vi "Create temperature log file.vi"(4 "path in":path) -> (0 "error out":errorcluster, 1 "refnum out":refnum<file>)   [LabVIEW 2022 SP3]
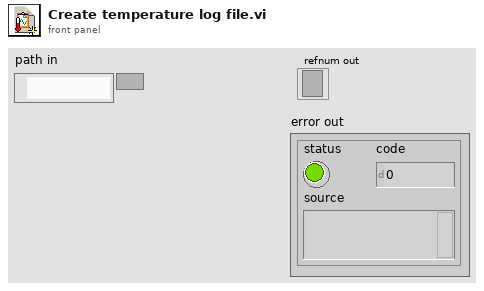
[diagram p1: front panel]
types:
  T1 = enum16{"open", "replace", "create", "open or create", "replace or create", "replace or create with confirmation"}
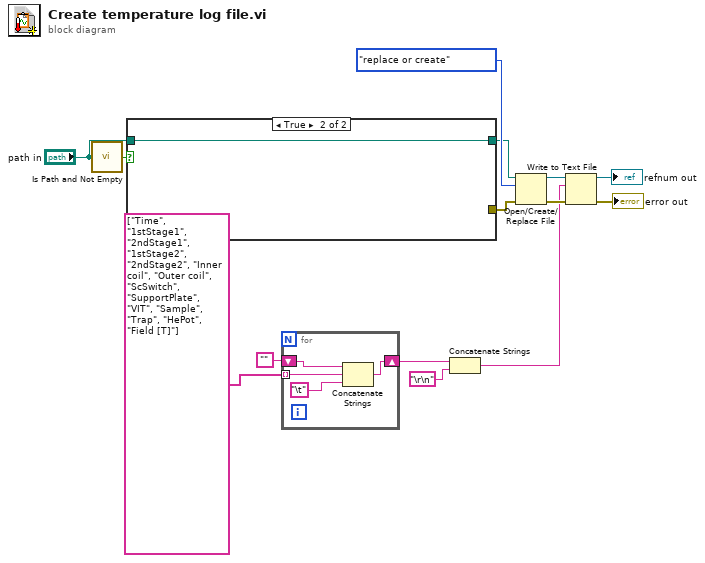
[diagram p0: block diagram]
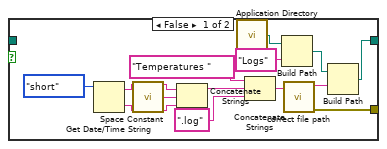
[diagram p2: hidden frame]
diagram:
  n1 = call <vilib>:"Is Path and Not Empty.vi"("path"="path in") -> ("Is Path and Not Empty?"=w4:bool)  [unwired: 4 in]
  n2 = case shown="True" w4 {
    tunnel: [w23 w29] -> w13
    tunnel: "path in" -> [_ w29]
    tunnel: [w15 _] -> w1
    frame False {
      n3 = Get Date/Time String(date format (0)=enum16{"short", "long", "abbreviated"}."short") -> (date string=w25:string, time string=w16:string)  [unwired: 2 in]
      n4 = call <vilib>:"Space Constant.vi"() -> ("String"=w19:string)
      n5 = Concatenate Strings(w25, w19, w16) -> (w20:string)
      n6 = call <vilib>:"Application Directory.vi"() -> ("Application Directory"=w21:path)
      n7 = Concatenate Strings("Temperatures " ("string"), w20, ".log" ("string")) -> (w17:string)
      n8 = Build Path(base path=w21, name or relative path="Logs") -> (appended path=w24:path)
      n9 = call "correct file path.vi"("input path"=w17) -> ("error out"=w15:errorcluster, "corrected path"=w18:string)  [unwired: 9 in]
      n10 = Build Path(base path=w24, name or relative path=w18) -> (appended path=w23:path)
    }
    frame True {
    }
  }
  n11 = for {
    tunnel: string[] ["Time", "1stStage1", "2ndStage1", "1stStage2", "2ndStage2", "Inner coil", "Outer coil", "ScSwitch", "SupportPlate", "VIT", "Sample", "Trap", "HePot", "Field [T]"] -> [w33] mode=indexing
    shift-right: [w31] -> w10
    shift-left: "" -> [w30]
    n12 = Concatenate Strings(w30, w33, "\t") -> (w31:string)
  }
  n13 = Concatenate Strings(w10, "\r\n") -> (w9:string)
  n14 = Open/Create/Replace File(file path (use dialog)=w13, error in=w1, operation (0:open)=T1."replace or create") -> (refnum out=w12:refnum<file>, error out=w11:errorcluster)  [unwired: 3 in, 1 out]
  n15 = Write to Text File(file (use dialog)=w12, text=w9, error in=w11) -> (refnum out=→"refnum out":refnum<file>, error out=→"error out":errorcluster)  [unwired: 1 in, 1 out]
